vi "Read All Child Attributes.vi"(7 "Actor in":refnum<class "Actor.lvclass">) -> (2 "All Child Attributes":T1)   [LabVIEW 2020, in "jettl.lvlib"]
uses:
  jettl.lvlib
  Actor/Actor.lvclass
  All Child Attributes.ctl
  Attributes/Attributes.lvclass
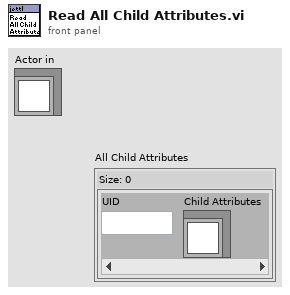
[diagram p1: front panel]
types:
  T1 = typedef "jettl.lvlib/All Child Attributes.ctl" = map{string, refnum<class "Attributes.lvclass">}
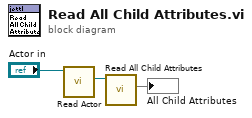
[diagram p0: block diagram]
diagram:
  n1 = call-dynamic "Read Actor.vi"("Actor in"="Actor in") -> ("Actor"=w3:refnum<class "Actor.lvclass">)  [unwired: 10 in]
  n2 = call-dynamic "Read All Child Attributes.vi"("Actor in"=w3) -> ("All Child Attributes"=→"All Child Attributes":T1)  [unwired: 10 in]
